vi "LVObject to JSON - Default - Pretty Print Disabled.vi"() -> ()   [LabVIEW 2017, in "Generic Object Serializer Tests.lvlib" / "Pretty Print.lvlib"]
uses:
  Pretty Print.lvlib
  Generic Object Serializer/Generic Object Serializer.lvclass
  <vilib>/addons/_JKI Toolkits/Caraya/classes/Assert/Assert Equal Value_Variant.vi
  <vilib>/addons/_JKI Toolkits/Caraya/classes/Test/Test.lvclass
  <vilib>/addons/_JKI Toolkits/Caraya/classes/Assert/Assert.lvclass
  Temperature Forecast/Temperature Forecast.lvclass
panel:
  out "error out":errorcluster
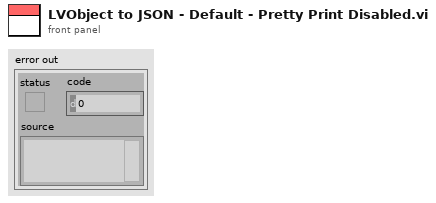
[diagram p1: front panel]
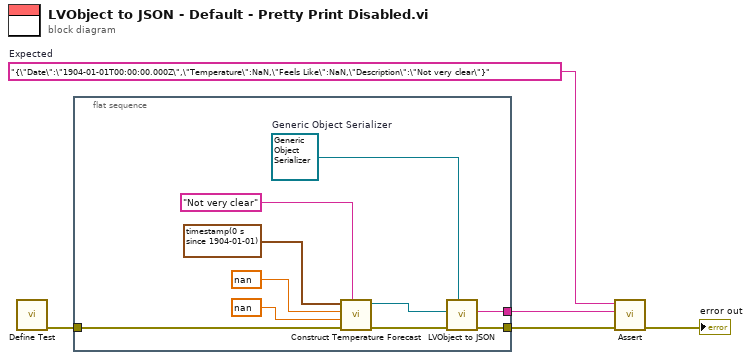
[diagram p0: block diagram]
diagram:
  w1 = "{\"Date\":\"1904-01-01T00:00:00.000Z\",\"Temperature\":NaN,\"Feels Like\":NaN,\"Description\":\"Not very clear\"}"  # Expected
  n1 = call <vilib>:"Define Test.vi"() -> ("error out"=w4:errorcluster)  [unwired: 11 in]
  n2 = flat-sequence {
    tunnel: w4 -> [w8]
    tunnel: [w14] -> w3
    tunnel: [w13] -> w2
    frame #0 {
      w15 = refnum<class "Generic Object Serializer.lvclass"> refnum  # Generic Object Serializer
      n3 = call "Construct Temperature Forecast.vi"("Description"="Not very clear", "error in (no error)"=w8, "Feels Like [°C]"=nan, "Temperature [°C]"=nan, "Date"=timestamp(0 s since 1904-01-01)) -> ("error out"=w7:errorcluster, "Temperature Forecast"=w6:refnum<class "Temperature Forecast.lvclass">)  [unwired: 5 in]
      n4 = call-dynamic "LVObject to JSON.vi"("LVClass Serializer"=w15, "error in (no error)"=w7, "Object"=w6) -> ("error out"=w14:errorcluster, "<JSON>Object"=w13:string)  [unwired: 7 in]
    }
  }
  n5 = call-poly <vilib>:"Assert.vi"("error in (no error)"=w3, "Y"=w2, "X"=w1) -> ("error out"=→"error out":errorcluster)  [unwired: 8 in]
